vi "rszvl Write Command.vi"(8 "error in (no error)":errorcluster, 10 "Command":string, 11 "VISA resource name":refnum<visa-resource-name>) -> (0 "error out":errorcluster, 3 "VISA resource name out":refnum<visa-resource-name>)   [LabVIEW 2014]
doc: "This VI sends a SCPI command to the instrument. Do not use this VI for queries (SCPI commands ending with the questiomark e.g. OUTPUT:STATE? )\nFor queries, use one of the following VIs:\n- Query ViBoolean.vi\n- Query ViInt32.vi\n- Query ViReal64.vi\n- Query ViString.vi\n- Query with OPC sync.vi"
uses:
  rszvl_rsidr_core.lvlib
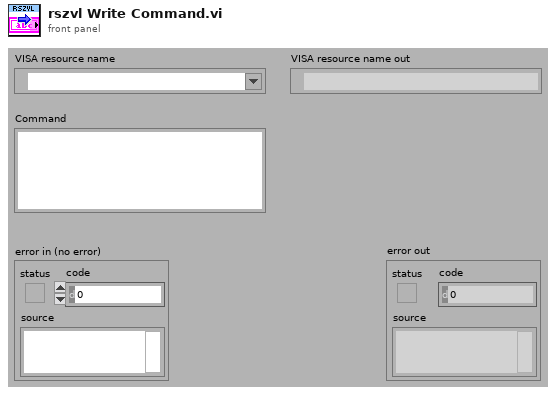
[diagram p1: front panel]
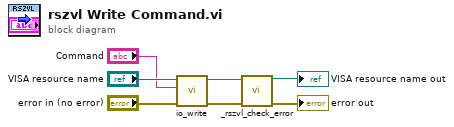
[diagram p0: block diagram]
diagram:
  n1 = call "io_write.vi"("error in"="error in (no error)", "write buffer"="Command", "VISA resource name"="VISA resource name") -> ("error out"=w5:errorcluster, "VISA resource name out"=w3:refnum<visa-resource-name>)  [unwired: 7 in]
  n2 = call "_rszvl_check_error.vi"("VISA resource name"=w3, "error in"=w5) -> ("VISA resource name out"=→"VISA resource name out":refnum<visa-resource-name>, "error out"=→"error out":errorcluster)  [unwired: 12 in]
